vi "Get Status.vi"(8 "error in (no error)":errorcluster, 11 "NI DMM in":refnum<class "NI DMM.lvclass">) -> (0 "error out":errorcluster, 2 "Status":variant, 3 "NI DMM out":refnum<class "NI DMM.lvclass">)   [LabVIEW 2020, in "NI DMM.lvlib" / "NI DMM.lvclass"]
uses:
  NI DMM.lvclass
  NI DMM.lvclass/NI DMM.ctl
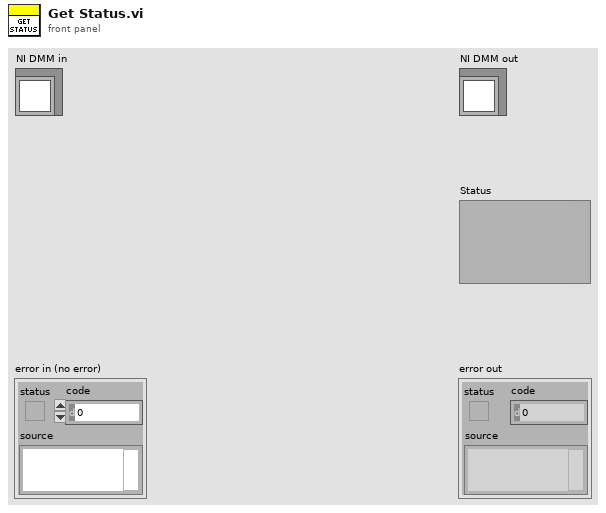
[diagram p1: front panel]
types:
  T1 = typedef "niDMM Acquisition State.ctl" = enum16{"Running", "Finished with Backlog", "Finished with no Backlog", "Paused", "No acquisition in progress"}
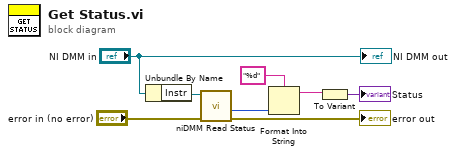
[diagram p0: block diagram]
diagram:
  n1 = Unbundle By Name("NI DMM in") -> ("Instr"=w7:refnum<k15>)
  n2 = call <instrlib>:"niDMM Read Status.vi"("error in (no error)"="error in (no error)", "instrument handle"=w7) -> ("error out"=→"error out":errorcluster, "Acquisition State"=w2:T1)  [unwired: 6 in, 2 out]
  n3 = Format Into String(format string="%d", w2) -> (resulting string=w3:string)  [unwired: 2 in, 1 out]
  n4 = To Variant(anything=w3) -> (Variant=→"Status":variant)
  "NI DMM out" <- "NI DMM in"
